vi "set_animal_id.vi"(4 "new animal ID":u16, 5 "old animal ID":u16, 6 "error in":errorcluster, 7 "setup ID":u16, 8 "settings array in":T2[](array[typedef]) {"stim ramp" min=1}, 9 "control cluster in":T1) -> (0 "error out":errorcluster={"status"=TRUE, "code"=1055, "source"="Property Node in setup_id_from_ctlref.vi->Untitled 1 (SubVI)"}, 1 "setup ID":u16, 2 "settings array out":T2[](array[typedef]) {"stim ramp" min=1}, 3 "control cluster out":T1)   [LabVIEW 2016]
uses:
  Type Definitions/vars_settings.ctl
  Type Definitions/stim_type.ctl
  Type Definitions/backlight_type.ctl
  Type Definitions/control_references.ctl
  <userlib>/_OpenG.lib/array/array.llb/Search 1D Array (U16)__ogtk.vi
  <userlib>/_OpenG.lib/array/array.llb/Delete Elements from 1D Array (U16)__ogtk.vi
  <userlib>/_OpenG.lib/array/array.llb/Filter 1D Array (U32)__ogtk.vi
  <userlib>/_OpenG.lib/array/array.llb/Conditional Auto-Indexing Tunnel (U32)__ogtk.vi
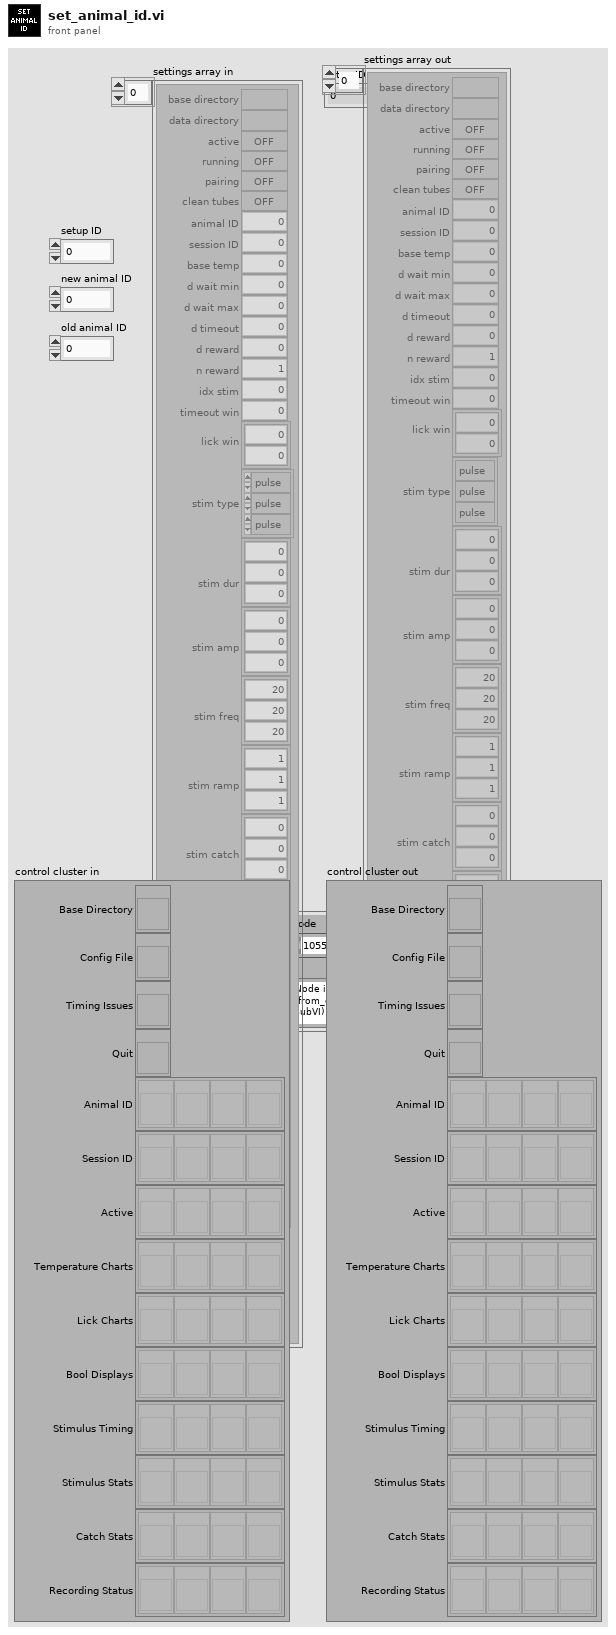
[diagram p1: front panel]
types:
  T1 = typedef "control_references.ctl" = cluster{"Base Directory":refnum<vi>, "Config File":refnum<vi>, "Timing Issues":refnum<vi>, "Quit":refnum<vi>, "Animal ID":refnum<vi>[], "Session ID":refnum<vi>[], "Active":refnum<vi>[], "Temperature Charts":refnum<vi>[], "Lick Charts":refnum<vi>[], "Bool Displays":refnum<vi>[], "Stimulus Timing":refnum<vi>[], "Stimulus Stats":refnum<vi>[], "Catch Stats":refnum<vi>[], "Recording Status":refnum<vi>[]}
  T2 = typedef "vars_settings.ctl" = cluster{"base directory":path, "data directory":path, "active":bool, "running":bool, "pairing":bool, "clean tubes":bool, "animal ID":u16, "session ID":u16, "base temp":dbl, "d wait min":u16, "d wait max":u16, "d timeout":u16, "d reward":u16, "n reward":u16, "idx stim":u16, "timeout win":u16, "lick win":i32[], "stim type":T3[], "stim dur":u16[], "stim amp":dbl[], "stim freq":u16[], "stim ramp":u16[], "stim catch":u8[], "square dur":u16[], "square delay":i16[], "square freq":u8[], "square dc":u8[], "stim shape":dbl[][], "square shape":bool[][], "backlight type":T4, "backlight freq":u16}
  T3 = typedef "stim_type.ctl" = enum16{"pulse", "vibration", "square", "sine"}
  T4 = typedef "backlight_type.ctl" = enum16{"none", "random", "regular"}
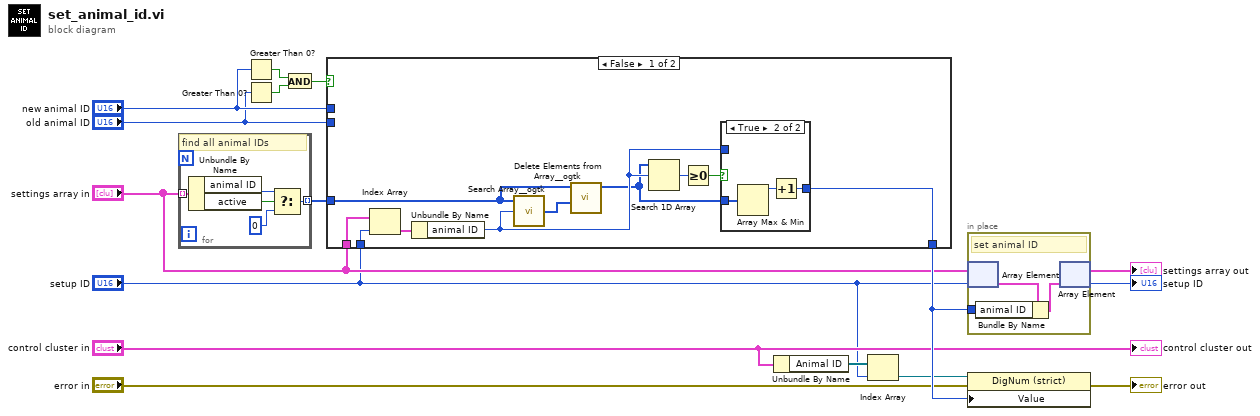
[diagram p0: block diagram]
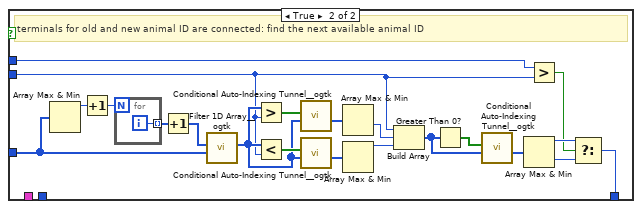
[diagram p3: hidden frame]
diagram:
  n1 = for {
    tunnel: "settings array in" -> [w21] mode=indexing
    tunnel: [w18] -> w16 mode=indexing
    # "find all animal IDs"
    n2 = Unbundle By Name(w21) -> ("animal ID"=w19:u16, "active"=w17:bool)
    n3 = Select(t=w19, s=w17, f=u16 0) -> (s? t:f=w18:u16)
  }
  n4 = Greater Than 0?(x="new animal ID") -> (x > 0?=w9:bool)
  n5 = Greater Than 0?(x="old animal ID") -> (x > 0?=w8:bool)
  n6 = And(x=w9, y=w8) -> (x .and. y?=w7:bool)
  n7 = case shown="False" w7 {
    tunnel: "new animal ID" -> [_ w44]
    tunnel: w16 -> [w23 w43]
    tunnel: "old animal ID" -> [_ w37]
    tunnel: [w29 w36] -> w14
    tunnel: "settings array in" -> [w28 _]
    tunnel: "setup ID" -> [w27 _]
    frame False {
      n8 = Index Array(array=w28, index=w27) -> (element=w26:T2)
      n9 = Unbundle By Name(w26) -> ("animal ID"=w24:u16)
      n10 = call-poly <userlib>:"Search Array__ogtk.vi"("Array"=w23, "Element Data"=w24) -> ("Indices of Elements"=w25:i32[])  [unwired: 7 in]
      n11 = call-poly <userlib>:"Delete Elements from Array__ogtk.vi"("indices"=w25, "array"=w23) -> ("array w/ subset deleted"=w22:u16[])  [unwired: 8 in, 1 out]
      n12 = Search 1D Array(1D array=w22, element=w24) -> (index of element=w31:i32)  [unwired: 1 in]
      n13 = Greater Or Equal To 0?(x=w31) -> (x >= 0?=w30:bool)
      n14 = case shown="True" w30 {
        tunnel: w22 -> [_ w35]
        tunnel: [w32 w33] -> w29
        tunnel: w24 -> [w32 _]
        frame False {
        }
        frame True {
          n15 = Array Max & Min(array=w35) -> (max value=w34:u16)  [unwired: 3 out]
          n16 = Increment(x=w34) -> (x+1=w33:u16)
        }
      }
    }
    frame True {
      # "terminals for old and new animal ID are connected: find the next available animal ID"
      n17 = Array Max & Min(array=w43) -> (max value=w56:u16)  [unwired: 3 out]
      n18 = Increment(x=w56) -> (x+1=w55:u16)
      n19 = for {
        N: w55 -> [_]
        tunnel: [w57] -> w54 mode=indexing
        i -> [w57]
      }
      n20 = Increment(x=w54) -> (x+1=w39:i32[])
      n21 = call-poly <userlib>:"Filter 1D Array__ogtk.vi"("items to filter"=w43, "array"=w39) -> ("filtered array"=w38:u32[])  [unwired: 4 in, 1 out]
      n22 = Greater?(x=w38, y=w37) -> (0:w53:bool[])
      n23 = Less?(x=w38, y=w37) -> (x < y?=w52:bool[])
      n24 = call-poly <userlib>:"Conditional Auto-Indexing Tunnel__ogtk.vi"("Array in"=w38, "Elements to keep"=w53) -> ("Filtered Array out"=w51:u32[])  [unwired: 5 in]
      n25 = call-poly <userlib>:"Conditional Auto-Indexing Tunnel__ogtk.vi"("Array in"=w38, "Elements to keep"=w52) -> ("Filtered Array out"=w50:u32[])  [unwired: 5 in]
      n26 = Array Max & Min(array=w51) -> (min value=w49:u32)  [unwired: 3 out]
      n27 = Array Max & Min(array=w50) -> (max value=w48:u32)  [unwired: 3 out]
      n28 = Build Array(w37, w49, w48) -> (w41:u32[])
      n29 = Greater Than 0?(x=w41) -> (x > 0?=w42:bool[])
      n30 = call-poly <userlib>:"Conditional Auto-Indexing Tunnel__ogtk.vi"("Array in"=w41, "Elements to keep"=w42) -> ("Filtered Array out"=w40:u32[])  [unwired: 5 in]
      n31 = Array Max & Min(array=w40) -> (max value=w47:u32, min value=w46:u32)  [unwired: 2 out]
      n32 = Greater?(x=w44, y=w37) -> (0:w45:bool)
      n33 = Select(t=w47, s=w45, f=w46) -> (s? t:f=w36:u32)
    }
  }
  n34 = Unbundle By Name("control cluster in") -> ("Animal ID"=w10:refnum<vi>[])
  n35 = Index Array(array=w10, index="setup ID") -> (element=w1:refnum<vi>)
  n36 = in-place {
    in-place-border: w14 -> [w59]
    # "set animal ID"
    n37 = in-place-array #1("settings array in", "setup ID") -> (w60:T2)
    n38 = Bundle By Name(cluster=w60, "animal ID"=w59) -> (w58:T2)
    n39 = in-place-array #1(w58) -> (→"settings array out":T2[], →"setup ID":i32)
  }
  n40 = property class="DigNum (strict)"(reference=w1, error in="error in", "Value"=w14) -> (error out=→"error out":errorcluster)  [unwired: 1 out]
  "control cluster out" <- "control cluster in"
